vi "GT 2D Compare Status.vi"(0 "cardNum":i16, 1 "chn":i16, 2 "pStatus":i16, 3 "pCount":i32, 4 "pFifo":i16, 5 "pFifoCount":i16, 6 "pBufCount":i16, 7 "error in (no error)":errorcluster caption="错误输入（无错误）") -> (20 "function return":i16, 22 "pStatus out":i16, 23 "pCount out":i32, 24 "pFifo out":i16, 25 "pFifoCount out":i16, 26 "pBufCount out":i16, 27 "error out":errorcluster caption="错误输出")   [LabVIEW 2014, in "gts.lvlib"]
doc: "GT_API GT_2DCompareStatus(short cardNum,short chn,short *pStatus,long *pCount,short *pFifo,short *pFifoCount,short *pBufCount =NULL);"
uses:
  gts.lvlib
  gts.dll
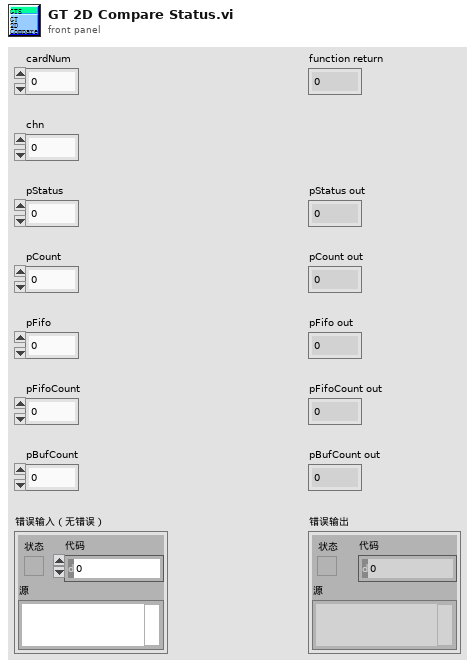
[diagram p1: front panel]
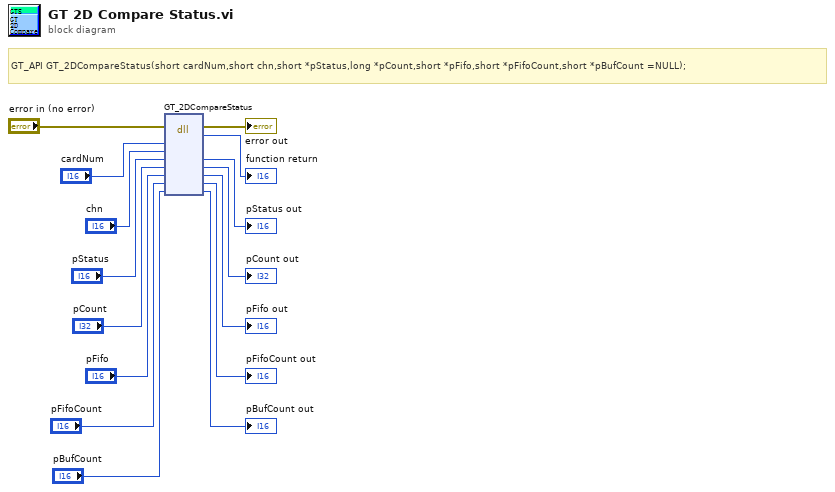
[diagram p0: block diagram]
diagram:
  # "GT_API GT_2DCompareStatus(short cardNum,short chn,short *pStatus,long *pCount,short *pFifo,short *pFifoCount,short *pBufCount =NULL);"
  n1 = dll-call lib="PTH2>abs F.多卡库-控制卡基本运动例程(labview)gts.*" fn="GT_2DCompareStatus"(error in="error in (no error)", "cardNum"="cardNum", "chn"="chn", "pStatus"="pStatus", "pCount"="pCount", "pFifo"="pFifo", "pFifoCount"="pFifoCount", "pBufCount"="pBufCount") -> (error out=→"error out":errorcluster, →"function return":i16, "pStatus"=→"pStatus out":i16, "pCount"=→"pCount out":i32, "pFifo"=→"pFifo out":i16, "pFifoCount"=→"pFifoCount out":i16, "pBufCount"=→"pBufCount out":i16)  [unwired: 4 in, 1 out]
